vi "Pico_Start Position.vi"(10 "Start Position":i32, 11 "Motor":i32) -> ()   [LabVIEW 2013]
uses:
  C:/Program Files/National Instruments/LabVIEW 2013/instr.lib/Newport_pico/Model 8742/LabVIEW 2009/CmdLib.dll
  Program Files/National Instruments/LabVIEW 2013/instr.lib/Newport_pico/Model 8742/LabVIEW 2009/CmdLib.dll
panel:
  out "Device Address Out":i32
  out "DeviceKey Out":string
  out "CmdLib Out":refnum<k24>
  out "Identification":string
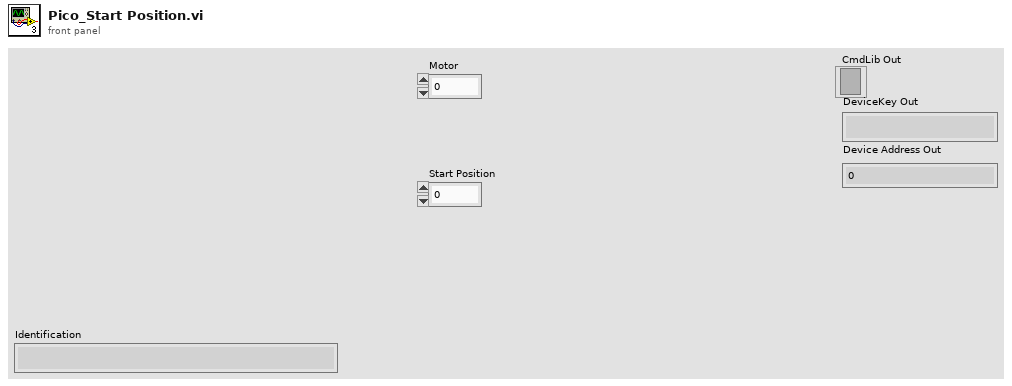
[diagram p1: front panel]
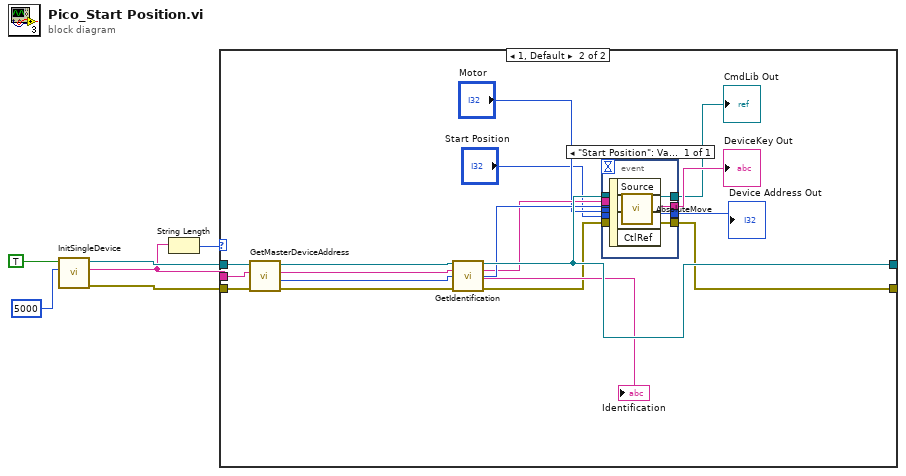
[diagram p0: block diagram]
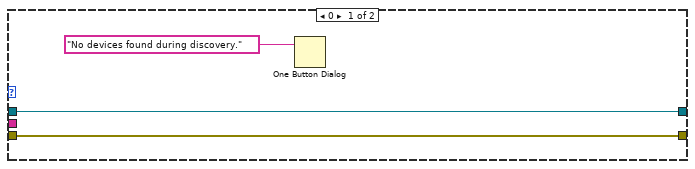
[diagram p2: hidden frame]
diagram:
  n1 = call <instrlib>:"InitSingleDevice.vi"("msecDelayForDiscovery"=5000, "logging"=TRUE) -> ("error out"=w2:errorcluster, "DeviceKey Out"=w1:string, "CmdLib Out"=w3:refnum<k24>)  [unwired: 3 in]
  n2 = String Length(string=w1) -> (length=w4:i32)
  n3 = case shown="1, Default" w4 {
    tunnel: [w9 w20] -> _
    tunnel: [w8 w13] -> _
    tunnel: w3 -> [w9 w27]
    tunnel: w2 -> [w8 w25]
    tunnel: w1 -> [_ w26]
    frame 0 {
      n4 = One Button Dialog(message="No devices found during discovery.") -> ()  [unwired: 1 in, 1 out]
    }
    frame 1, Default {
      n5 = call <instrlib>:"GetMasterDeviceAddress.vi"("error in (no error)"=w25, "DeviceKey In"=w26, "CmdLib In"=w27) -> ("error out"=w24:errorcluster, "Device Address"=w21:i32, "DeviceKey Out"=w22:string, "CmdLib Out"=w23:refnum<k24>)  [unwired: 1 in]
      n6 = call <instrlib>:"GetIdentification.vi"("CmdLib In"=w23, "DeviceKey In"=w22, "Device Address In"=w21, "error in (no error)"=w24) -> ("CmdLib Out"=w20:refnum<k24>, "DeviceKey Out"=w17:string, "Device Address Out"=w18:i32, "Identification"=→"Identification":string, "error out"=w14:errorcluster)  [unwired: 7 in]
      n7 = event shown="[0] \"Start Position\": Value Change" {
        selector: _ -> [_]
        dyn-events: _ -> [_]
        timeout: _ -> [_]
        tunnel: w20 -> [w37]
        tunnel: w18 -> [w36]
        tunnel: w17 -> [w35]
        tunnel: "Motor" -> [w34]
        tunnel: "Start Position" -> [w33]
        tunnel: w14 -> [w32]
        tunnel: [w31] -> w13
        tunnel: [w30] -> w10
        tunnel: [w29] -> w12
        tunnel: [w28] -> w11
        event "Start Position": Value Change {
          n8 = event-data() -> ()  [unwired: 1 in, 4 out]
          n9 = call <instrlib>:"AbsoluteMove.vi"("CmdLib In"=w37, "DeviceKey In"=w35, "Device Address In"=w36, "Motor"=w34, "Target Pos"=w33, "error in (no error)"=w32) -> ("CmdLib Out"=w30:refnum<k24>, "DeviceKey Out"=w29:string, "Device Address Out"=w28:i32, "error out"=w31:errorcluster)  [unwired: 10 in]
        }
      }
      "CmdLib Out" <- w10
      "DeviceKey Out" <- w12
      "Device Address Out" <- w11
    }
  }
